vi "Cubic Spline Fit.vi"(0 "Y":dbl[](array[numeric]), 5 "X":dbl[](array[numeric]), 7 "Weight":dbl[](array[numeric]) format="%#.6g", 9 "balance parameter":dbl=-1.0, 11 "Smoothness":dbl[](array[numeric])) -> (4 "Best Cubic Spline Fit":dbl[](array[numeric]), 15 "error":i32)   [LabVIEW 2020, in "NI_AALPro.lvlib"]
doc: "Uses cubic spline fitting to smooth a data set (<B>X</B>, <B>Y</B>) according to the <B>balance parameter</B>."
uses:
  <vilib>/Analysis/NI_AALPro.lvlib
  <resource>/lvanlys.dll
panel:
  # "Cubic Spline Fit"
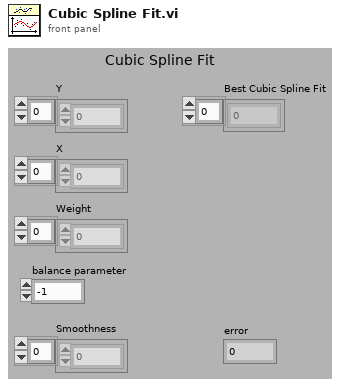
[diagram p1: front panel]
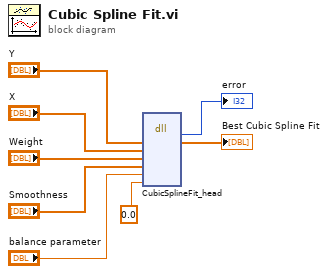
[diagram p0: block diagram]
diagram:
  n1 = dll-call lib="e:/builds/penguin/labview/branches/2020/dev/dist/resource/lvanlys.*" fn="CubicSplineFit_head"("y"="Y", "x"="X", "weight"="Weight", "lambda"="Smoothness", "p"="balance parameter", "merit"=0.0) -> (→"error":i32, "y"=→"Best Cubic Spline Fit":dbl[])  [unwired: 8 in, 2 out]
